vi "close pointers.vi"(7 "HasoData in":refnum<class "HasoData.lvclass">, 8 "error in (no error)":errorcluster, 9 "Phase in":refnum<class "Phase.lvclass">, 10 "ComputePhaseSet.lvclass in":refnum<class "ComputePhaseSet.lvclass">, 11 "Pupil in":refnum<class "Pupil.lvclass">) -> (0 "error out":errorcluster)   [LabVIEW 2020, in "HASO4_3.lvclass"]
uses:
  HASO4_3.lvclass
  WaveKit/Classes/ComputePhaseSet/ComputePhaseSet.lvclass
  WaveKit/Classes/HasoData/HasoData.lvclass
  WaveKit/Classes/Pupil/Pupil.lvclass
  WaveKit/Classes/Phase/Phase.lvclass
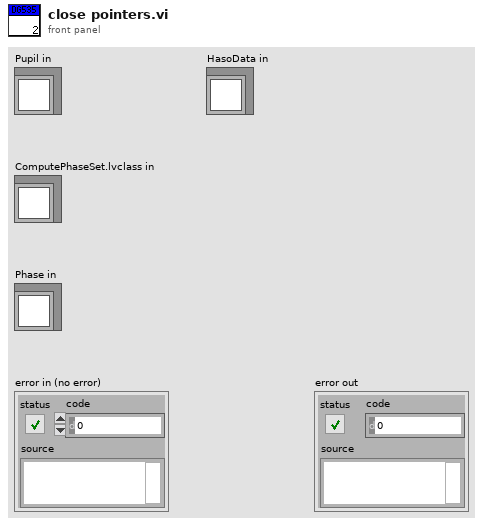
[diagram p1: front panel]
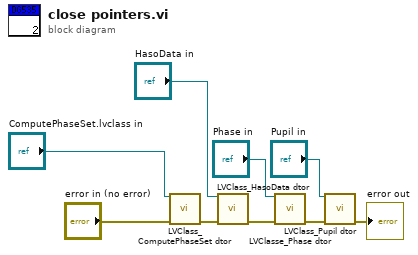
[diagram p0: block diagram]
diagram:
  n1 = call "LVClass_ComputePhaseSet dtor.vi"("ComputePhaseSet in"="ComputePhaseSet.lvclass in", "error in (no error)"="error in (no error)") -> ("error out"=w7:errorcluster)  [unwired: 12 in, 1 out]
  n2 = call "LVClass_HasoData dtor.vi"("HasoData in"="HasoData in", "error in (no error)"=w7) -> ("error out"=w9:errorcluster)  [unwired: 12 in, 1 out]
  n3 = call "LVClasse_Phase dtor.vi"("Phase in"="Phase in", "error in (no error)"=w9) -> ("error out"=w3:errorcluster)  [unwired: 12 in, 1 out]
  n4 = call "LVClass_Pupil dtor.vi"("Pupil in"="Pupil in", "error in (no error)"=w3) -> ("error out"=→"error out":errorcluster)  [unwired: 12 in, 1 out]
